vi "Save_TDMS.vi"(0 "Voltage":dbl, 1 "Current":dbl, 2 "Resistance":dbl, 3 "Temperature":dbl, 4 "u_A(temp)":dbl, 5 "TDMS IN":refnum<k34>, 7 "Timestamp":timestamp) -> (19 "TDMS OUT":refnum<k34>)   [LabVIEW 2022 SP3]
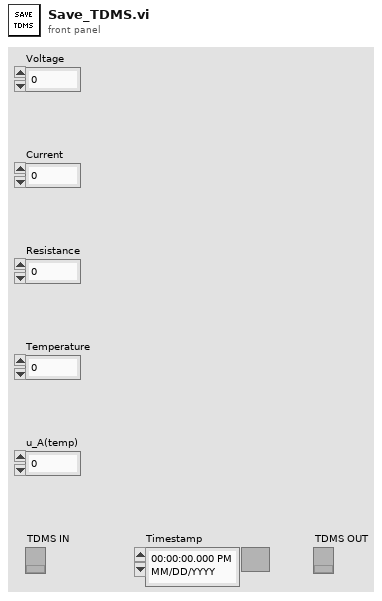
[diagram p1: front panel]
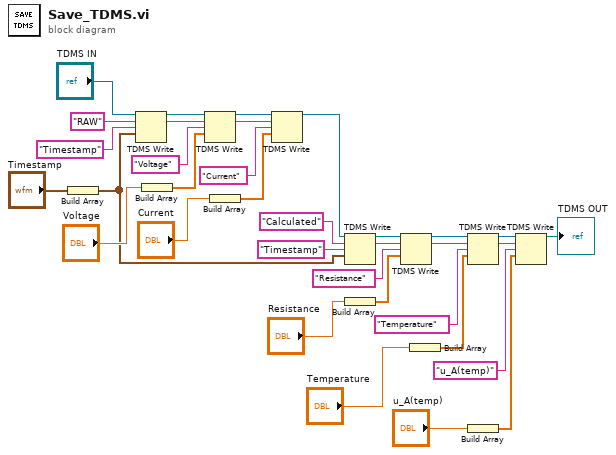
[diagram p0: block diagram]
diagram:
  n1 = Build Array("Timestamp") -> (w8:timestamp[])
  n2 = TDMS Write(0:"TDMS IN", 5:"RAW" ("group name in (Untitled)"), 7:"Timestamp" ("group name in (Untitled)"), 9:w8) -> (4:w31:refnum<k34>, 6:w29:string)  [unwired: 2 in, 2 out]
  n3 = Build Array("Voltage") -> (w27:dbl[])
  n4 = TDMS Write(0:w31, 5:w29, 7:"Voltage", 9:w27) -> (4:w25:refnum<k34>, 6:w24:string)  [unwired: 2 in, 2 out]
  n5 = Build Array("Current") -> (w21:dbl[])
  n6 = TDMS Write(0:w25, 5:w24, 7:"Current", 9:w21) -> (4:w20:refnum<k34>)  [unwired: 2 in, 3 out]
  n7 = TDMS Write(0:w20, 5:"Calculated" ("group name in (Untitled)"), 7:"Timestamp" ("group name in (Untitled)"), 9:w8) -> (4:w18:refnum<k34>, 6:w15:string)  [unwired: 2 in, 2 out]
  n8 = Build Array("Resistance") -> (w7:dbl[])
  n9 = TDMS Write(0:w18, 5:w15, 7:"Resistance" ("group name in (Untitled)"), 9:w7) -> (4:w17:refnum<k34>, 6:w14:string)  [unwired: 2 in, 2 out]
  n10 = Build Array("Temperature") -> (w4:dbl[])
  n11 = TDMS Write(0:w17, 5:w14, 7:"Temperature" ("group name in (Untitled)"), 9:w4) -> (4:w16:refnum<k34>, 6:w13:string)  [unwired: 2 in, 2 out]
  n12 = Build Array("u_A(temp)") -> (w2:dbl[])
  n13 = TDMS Write(0:w16, 5:w13, 7:"u_A(temp)" ("group name in (Untitled)"), 9:w2) -> (4:→"TDMS OUT":refnum<k34>)  [unwired: 2 in, 3 out]
